vi "Get Active Project Name.vi"(8 "error in":errorcluster) -> (0 "error out":errorcluster, 2 "Project Name":string, 3 "Project Ref":refnum<vi>)   [LabVIEW 2020, in "Panter Dashboard.lvlib"]
uses:
  Panter Dashboard.lvlib
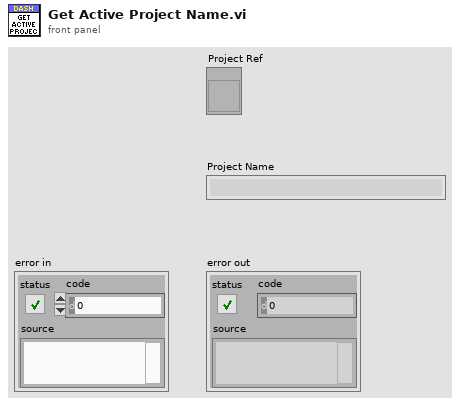
[diagram p1: front panel]
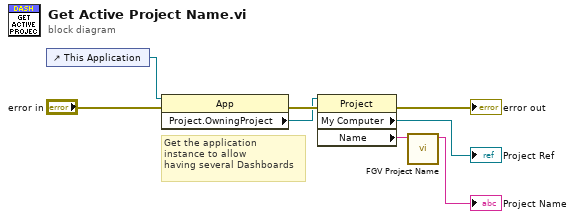
[diagram p0: block diagram]
diagram:
  # "Get the application\ninstance to allow\nhaving several Dashboards"
  n1 = control-ref of="This Application"() -> (w4:refnum<vi>)
  n2 = property class="App"(reference=w4, error in="error in") -> (error out=w7:errorcluster, "Project.OwningProject"=w5:refnum<vi>)  [unwired: 1 out]
  n3 = property class="Project"(reference=w5, error in=w7) -> (error out=→"error out":errorcluster, "My Computer"=→"Project Ref":refnum<vi>, "Name"=w2:string)  [unwired: 1 out]
  n4 = call "FGV Project Name.vi"("Project Name"=w2) -> ("Project Name Out"=→"Project Name":string)  [unwired: 10 in]
